vi "Close Refnum.vi"(8 "Error In":errorcluster, 11 "Add In":refnum<class "Add.lvclass">) -> (0 "Error Out":errorcluster, 3 "Add Out":refnum<class "Add.lvclass">)   [LabVIEW 2021, in "Calculator.lvlib" / "Add.lvclass"]
doc: "This VI is a overriding method that closes the subpanel reference."
uses:
  Add.lvclass
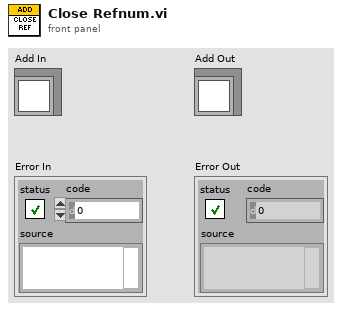
[diagram p1: front panel]
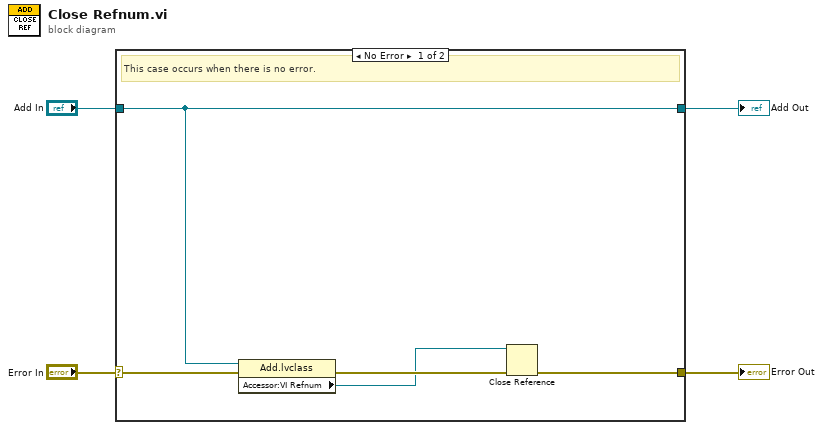
[diagram p0: block diagram]
diagram:
  n1 = case shown="No Error" "Error In" {
    selector: "Error In" -> [w6 w11]
    tunnel: [w8 w11] -> w3
    tunnel: [w5 w10] -> w1
    tunnel: "Add In" -> [w5 w10]
    frame No Error {
      # "This case occurs when there is no error."
      n2 = property class="Add.lvclass"(reference=w5, error in=w6) -> (error out=w9:errorcluster, "Accessor:VI Refnum"=w7:refnum<vi>)  [unwired: 1 out]
      n3 = Close Reference(reference=w7, error in (no error)=w9) -> (error out=w8:errorcluster)
    }
    frame Error {
      # "This case occurs if there is any error."
    }
  }
  "Error Out" <- w3
  "Add Out" <- w1
